vi "Varianta 1.vi"() -> ()   [LabVIEW 2024]
uses:
  <vilib>/picture/picture.llb/imagedata.ctl
panel:
  out "?":bool
  out "Tipul piesei":string
  out "new picture":picture
  out "image data":T1
  in  "Path":path
  # "este buna piesa?"
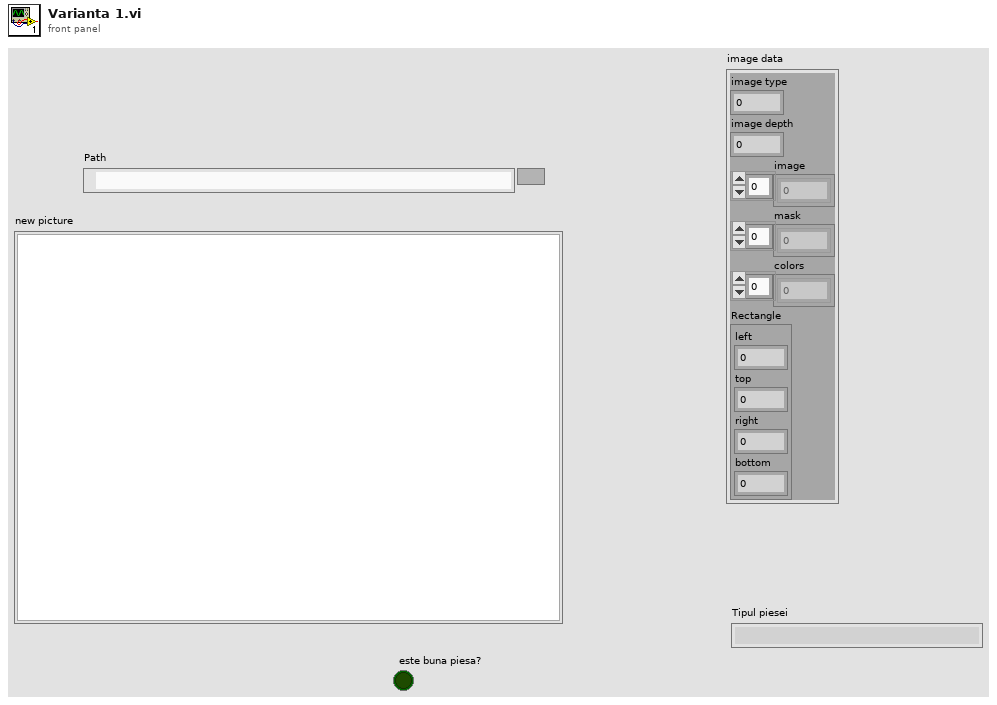
[diagram p1: front panel]
types:
  T1 = typedef "imagedata.ctl" = cluster{"image type":i32, "image depth":i32, "image":u8[], "mask":u8[], "colors":u32[], "Rectangle":cluster{"left":i16, "top":i16, "right":i16, "bottom":i16}}
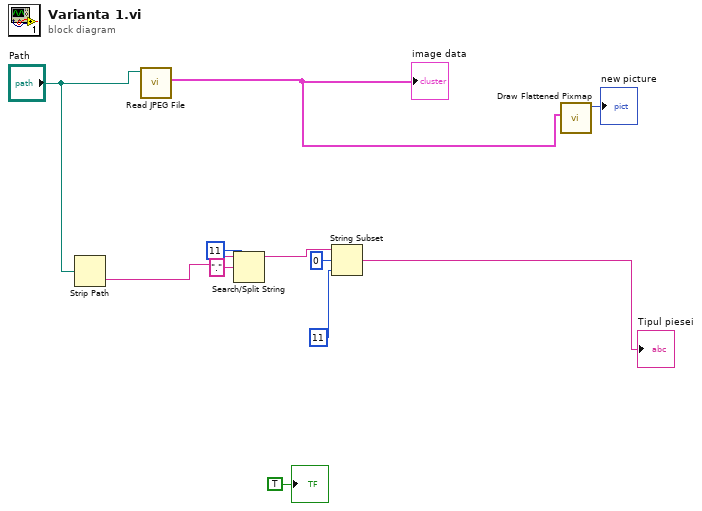
[diagram p0: block diagram]
diagram:
  n1 = Strip Path(path="Path") -> (name=w8:string)  [unwired: 1 out]
  n2 = call <vilib>:"Read JPEG File.vi"("path to JPEG file"="Path") -> ("image data"=w11:T1)  [unwired: 8 in, 2 out]
  "image data" <- w11
  n3 = Search/Split String(string=w8, search string/char (-)=".", offset (0)=11) -> (substring before match=w5:string)  [unwired: 2 out]
  n4 = String Subset(string=w5, offset (0)=0, length (rest)=11 ("length (rest)")) -> (substring=→"Tipul piesei":string)
  n5 = call <vilib>:"Draw Flattened Pixmap.vi"("image data"=w11) -> ("new picture"=→"new picture":picture)  [unwired: 8 in]
  "?" <- TRUE ("Boolean")
